vi "Do.vi"(8 "error in (no error)":errorcluster, 10 "Actor in":refnum<class "Actor.lvclass">, 11 "FlushAckMsg":refnum<class "FlushAckMsg.lvclass">) -> (0 "error out":errorcluster, 2 "Actor out":refnum<class "Actor.lvclass">)   [LabVIEW 2026, in "Lumberjack.lvlib" / "FlushAckMsg.lvclass"]
doc: "<p>(<strong>Filename</strong>: <span class=\"dnl\">Actor Framework.lvlib:Message.lvclass:Do.vi</span>)</p>\n<p>Defines what a message does when it is received by an actor. Generally, a message instructs an actor to invoke one of its methods. By default, this method does nothing. A child class must override it to define behavior.</p>"
uses:
  FlushAckMsg.lvclass
  <vilib>/ActorFramework/Actor/Actor.lvclass
  FlushAckMsg.lvclass/FlushAckMsg.ctl
  LogManager/LogManager.lvclass/LogManager.lvclass
  C:/Program Files (x86)/National Instruments/LabVIEW 2026/vi.lib/ActorFramework/Actor/Actor.lvclass
  C:/Users/dallis/OneDrive - Velico Medical/Documents/Personal/LabVIEW Coding Projects/Lumberjack/src/Core/LogManager/LogManager.lvclass/LogManager.lvclass
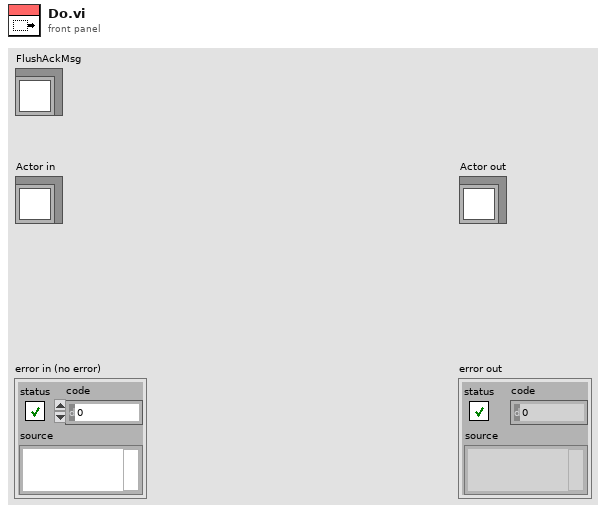
[diagram p1: front panel]
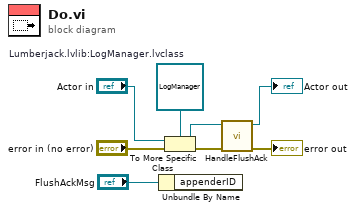
[diagram p0: block diagram]
diagram:
  w2 = refnum<class "LogManager.lvclass"> refnum  # Lumberjack.lvlib:LogManager.lvclass
  n1 = Unbundle By Name("FlushAckMsg") -> ()  [unwired: 1 out]
  n2 = To More Specific Class(target class=w2, reference="Actor in", error in="error in (no error)") -> (specific class reference=w4:refnum<class "LogManager.lvclass">, error out=w5:errorcluster)
  n3 = call "HandleFlushAck.vi"("error in (no error)"=w5, "LogManager in"=w4) -> ("error out"=→"error out":errorcluster, "LogManager out"=→"Actor out":refnum<class "LogManager.lvclass">)  [unwired: 8 in]
